vi "Labview Demo 1.vi"() -> ()   [LabVIEW 2016]
uses:
  C:/Program Files (x86)/Doodlebase/Transformer/Schemaport.Doodlebase.Transformer.dll
  Program Files (x86)/Doodlebase/Transformer/Schemaport.Doodlebase.Transformer.dll
panel:
  out "Network Success":bool
  in  "Variables":dbl
  in  "File Path Directory":path
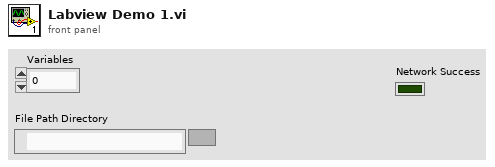
[diagram p1: front panel]
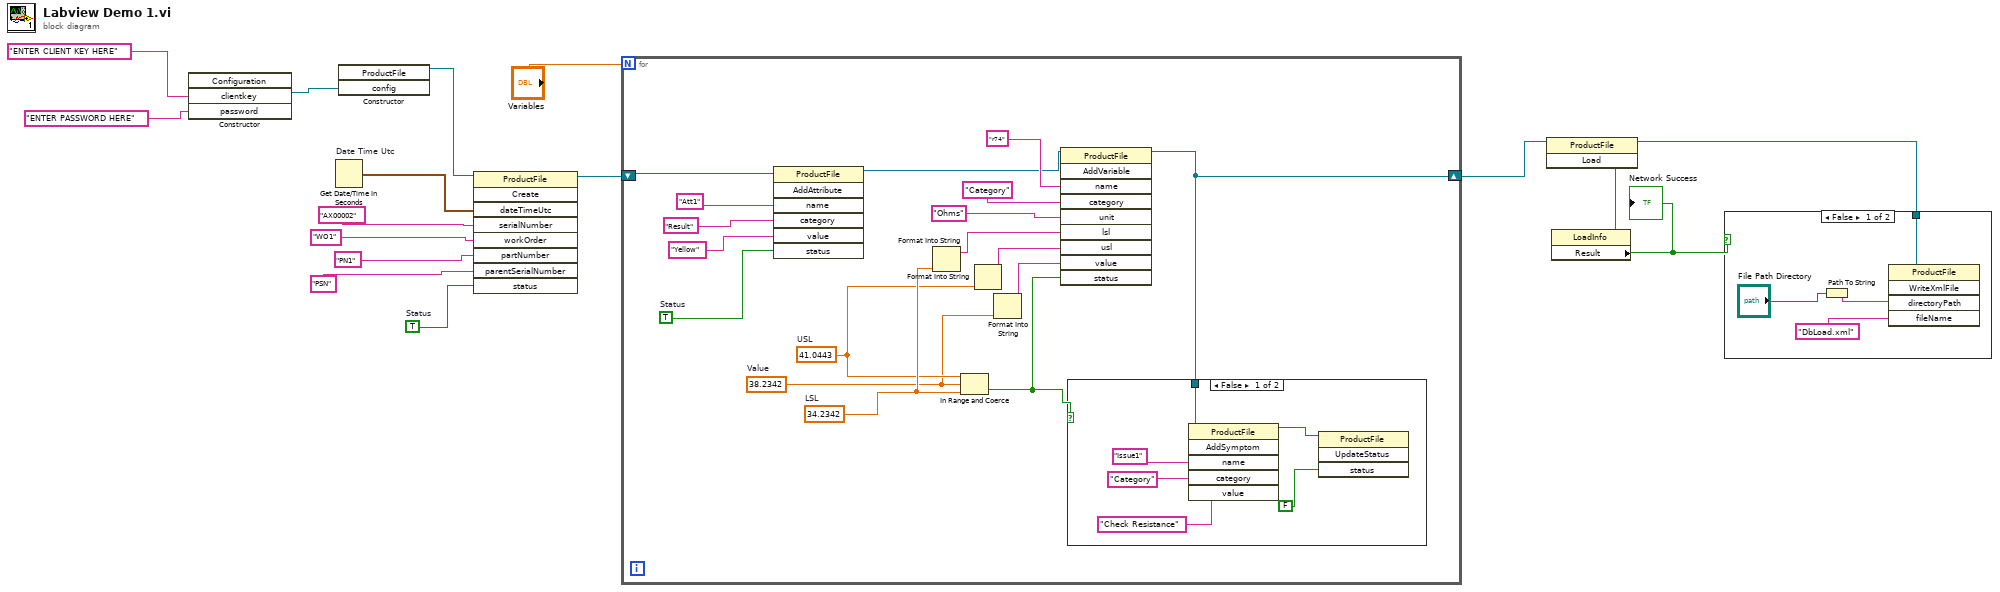
[diagram p0: block diagram]
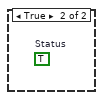
[diagram p3: hidden frame]
diagram:
  w10 = TRUE  # Status
  n1 = constructor class="Configuration"("clientkey"="ENTER CLIENT KEY HERE", "password"="ENTER PASSWORD HERE") -> (reference out=w7:refnum<k24>)  [unwired: 3 in, 4 out]
  n2 = Get Date/Time In Seconds "Date Time Utc"() -> (seconds since 1Jan1904=w9:timestamp)
  n3 = constructor class="ProductFile"("config"=w7) -> (reference out=w14:refnum<k24>)  [unwired: 3 in, 3 out]
  n4 = invoke class="ProductFile" method="Create"(reference=w14, "dateTimeUtc"=w9, "serialNumber"="AX00002", "workOrder"="WO1", "partNumber"="PN1", "parentSerialNumber"="PSN", "status"=w10) -> (reference out=w8:refnum<k24>)  [unwired: 2 in, 8 out]
  n5 = for {
    N: "Variables" -> [_]
    shift-right: [w18] -> w1
    shift-left: w8 -> [w33]
    w24 = 34.2342  # LSL
    w22 = 41.0443  # USL
    w19 = 38.2342  # Value
    w29 = TRUE  # Status
    n6 = invoke class="ProductFile" method="AddAttribute"(reference=w33, "name"="Att1", "category"="Result", "value"="Yellow", "status"=w29) -> (reference out=w17:refnum<k24>)  [unwired: 2 in, 6 out]
    n7 = Format Into String(w24) -> (resulting string=w23:string)  [unwired: 3 in, 1 out]
    n8 = In Range and Coerce(upper limit=w22, x=w19, lower limit=w24) -> (In Range?=w25:bool)  [unwired: 1 out]
    n9 = Format Into String(w22) -> (resulting string=w21:string)  [unwired: 3 in, 1 out]
    n10 = Format Into String(w19) -> (resulting string=w20:string)  [unwired: 3 in, 1 out]
    n11 = invoke class="ProductFile" method="AddVariable"(reference=w17, "name"="r74", "category"="Category", "unit"="Ohms", "lsl"=w23, "usl"=w21, "value"=w20, "status"=w25) -> (reference out=w18:refnum<k24>)  [unwired: 2 in, 9 out]
    n12 = case shown="False" w25 {
      tunnel: w18 -> [w36 _]
      frame False {
        n13 = invoke class="ProductFile" method="AddSymptom"(reference=w36, "name"="Issue1", "category"="Category", "value"="Check Resistance") -> (reference out=w34:refnum<k24>)  [unwired: 2 in, 5 out]
        n14 = invoke class="ProductFile" method="UpdateStatus"(reference=w34, "status"=FALSE) -> ()  [unwired: 2 in, 4 out]
      }
      frame True {
        (unwired) TRUE  # Status
      }
    }
  }
  n15 = invoke class="ProductFile" method="Load"(reference=w1) -> (reference out=w2:refnum<k24>, "Load"=w3:refnum<k24>)  [unwired: 2 in, 1 out]
  n16 = property class="LoadInfo"(reference=w3) -> ("Result"=w5:bool)  [unwired: 1 in, 2 out]
  "Network Success" <- w5
  n17 = case shown="False" w5 {
    tunnel: w2 -> [w41 _]
    frame False {
      n18 = Path To String(path="File Path Directory") -> (string=w42:string)
      n19 = invoke class="ProductFile" method="WriteXmlFile"(reference=w41, "directoryPath"=w42, "fileName"="DbLoad.xml") -> ()  [unwired: 2 in, 5 out]
    }
    frame True {
    }
  }
